vi "eventToClient.vi"(8 "error in (no error)":errorcluster, 10 "eventConnID":T1, 11 "TcpServer in":refnum<class "TcpServer.lvclass">) -> (0 "error out":errorcluster, 3 "TcpServer out":refnum<class "TcpServer.lvclass">)   [LabVIEW 2018, in "TcpServer.lvclass"]
doc: "Send an Event to the TCP Client."
uses:
  TcpServer.lvclass
  typedef/eventConnIDTypeDef.ctl
  typedef/packetConnIDTypeDef.ctl
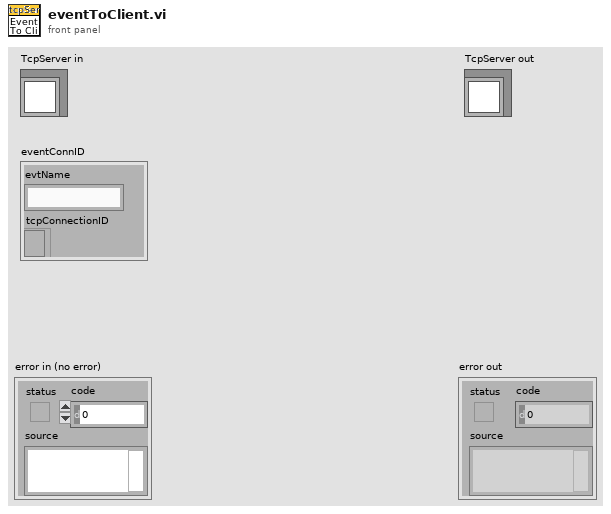
[diagram p1: front panel]
types:
  T1 = typedef "TcpServer.lvclass/eventConnIDTypeDef.ctl" = cluster{"evtName":string, "tcpConnectionID":refnum<k5>}
  T2 = typedef "TcpServer.lvclass/packetConnIDTypeDef.ctl" = cluster{"packet":string, "tcpConnectionID":refnum<k5>, "firstCmdId":bool}
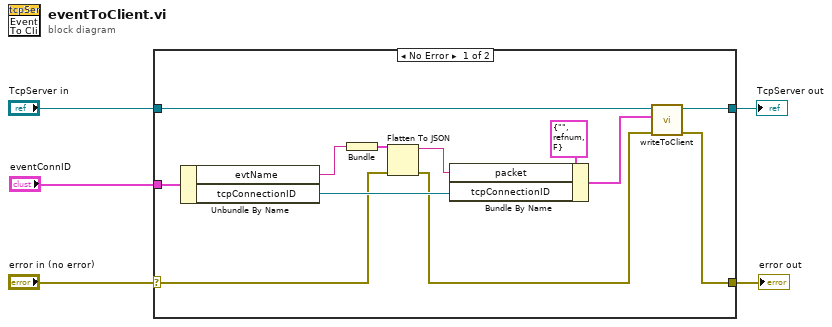
[diagram p0: block diagram]
diagram:
  n1 = case shown="No Error" "error in (no error)" {
    selector: "error in (no error)" -> [w7 w19]
    tunnel: [w15 w19] -> w4
    tunnel: [w16 w18] -> w2
    tunnel: "TcpServer in" -> [w17 w18]
    tunnel: "eventConnID" -> [w13 _]
    frame No Error {
      n2 = Unbundle By Name(w13) -> ("evtName"=w12:string, "tcpConnectionID"=w10:refnum<k5>)
      n3 = Bundle("evtName"=w12) -> (w14:cluster{"evtName":string})  [unwired: 1 in]
      n4 = Flatten To JSON(anything=w14, error in (no error)=w7) -> (JSON string=w9:string, 11:w8:errorcluster)  [unwired: 1 in]
      n5 = Bundle By Name(cluster=T2 {"packet"="", "tcpConnectionID"=refnum, "firstCmdId"=FALSE} ("packetConnID"), "packet"=w9, "tcpConnectionID"=w10) -> (w6:T2)
      n6 = call "writeToClient.vi"("error in (no error)"=w8, "packetConnID"=w6, "tcpServer in"=w17) -> ("error out"=w15:errorcluster, "tcpServer out"=w16:refnum<class "TcpServer.lvclass">)  [unwired: 7 in]
    }
    frame Error {
    }
  }
  "error out" <- w4
  "TcpServer out" <- w2
